vi "getLockedAttributes.vi"(8 "error in (no error)":errorcluster, 11 "IComponent in":refnum<class "IComponent.lvclass">) -> (0 "error out":errorcluster, 2 "locked Attributes out out":string[](array[string]), 3 "IComponent out":refnum<class "IComponent.lvclass">)   [LabVIEW 2022 SP3, in "openDAQ.lvlib" / "IBaseObject.lvlib" / "IPropertyObject.lvlib" / "IComponent.lvlib" / "IComponent.lvclass"]
uses:
  <instrlib>/openDAQ/Public/Classes/IComponent/IComponent.lvclass
  <instrlib>/openDAQ/Public/Classes/IComponent/IComponent.lvclass/IComponent.ctl
  <instrlib>/openDAQ/Public/Classes/daqCoreTypes/IList/IList.lvclass
  <instrlib>/openDAQ/Public/Classes/daqCoreTypes/IList/Polymorphic/getList/getStringList.vi
  <instrlib>/openDAQ/Binaries/Windows/x86/copendaq32.dll
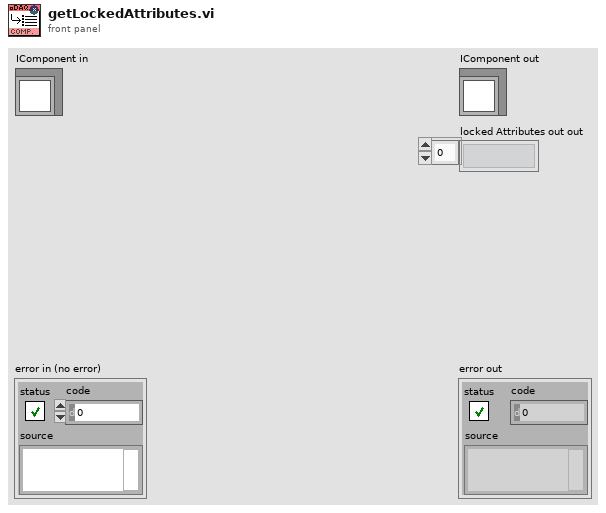
[diagram p1: front panel]
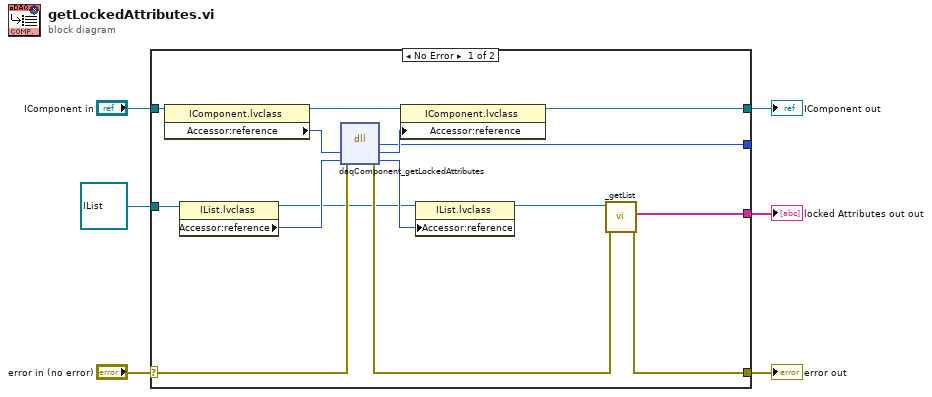
[diagram p0: block diagram]
diagram:
  n1 = case shown="No Error" "error in (no error)" {
    selector: "error in (no error)" -> [w20 w23]
    tunnel: [w12 w23] -> w5
    tunnel: [w9 w22] -> w3
    tunnel: "IComponent in" -> [w21 w22]
    tunnel: refnum<class "IList.lvclass"> refnum ("openDAQ.lvlib:daqCoreTypes.lvlib:IList.lvclass") -> [w19 _]
    tunnel: [w11 _] -> w1
    tunnel: [w7 _] -> _
    frame No Error {
      n2 = property class="IComponent.lvclass"(reference=w21) -> (reference out=w10:refnum<class "IComponent.lvclass">, "Accessor:reference"=w18:i64)  [unwired: 1 in, 1 out]
      n3 = property class="IList.lvclass"(reference=w19) -> (reference out=w8:refnum<class "IList.lvclass">, "Accessor:reference"=w17:i64)  [unwired: 1 in, 1 out]
      n4 = dll-call lib="C:/Program Files (x86)/National Instruments/LabVIEW 2022/instr.lib/openDAQ/Binaries/Windows/x86/copendaq*.*" fn="daqComponent_getLockedAttributes"(error in=w20, "component"=w18, "lockedAttributes"=w17) -> (error out=w13:errorcluster, "return type"=w7:u32, "component"=w16:i64, "lockedAttributes"=w15:i64)  [unwired: 2 in, 1 out]
      n5 = property class="IComponent.lvclass"(reference=w10, "Accessor:reference"=w16) -> (reference out=w9:refnum<class "IComponent.lvclass">)  [unwired: 1 in, 1 out]
      n6 = property class="IList.lvclass"(reference=w8, "Accessor:reference"=w15) -> (reference out=w14:refnum<class "IList.lvclass">)  [unwired: 1 in, 1 out]
      n7 = call-poly <instrlib>:"_getList.vi"("error in (no error)"=w13, "IList in"=w14) -> ("error out"=w12:errorcluster, "String List out"=w11:string[])  [unwired: 8 in]
    }
    frame Error {
    }
  }
  "error out" <- w5
  "IComponent out" <- w3
  "locked Attributes out out" <- w1
